vi "Initialize.vi"(6 "Interface":enum16{"RS232", "USB", "Ethernet"}(ring)=enum."USB", 8 "error in (no error)":errorcluster, 9 "reset":bool, 10 "ID query":bool=TRUE, 11 "Address":string) -> (0 "error out":errorcluster, 3 "VISA resource name out":refnum<visa-resource-name>)   [LabVIEW 2016, in "SR7270 Drivers.lvlib" / "SR7270 Drivers.lvclass"]
doc: "This VI passes the addressing information in the instrument decriptor to the Instr Open VI and returns the instrument ID. You can optionally reset the instrument by setting the front panel reset control. You must run this VI before using any of the instrument driver VIs for this instrument.\n\n12 May 2009: First Release"
uses:
  SR7270 Drivers.lvclass
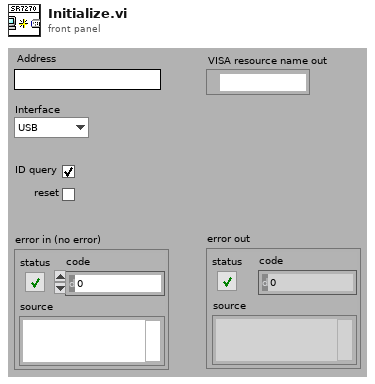
[diagram p1: front panel]
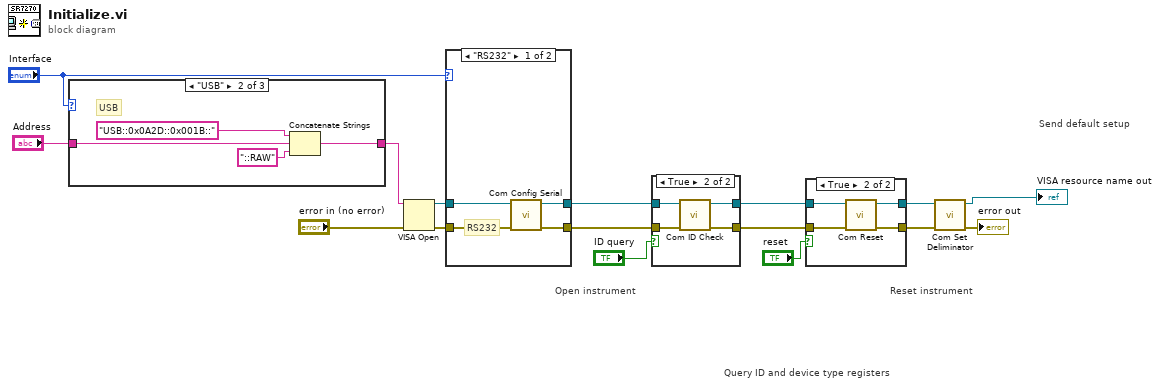
[diagram p0: block diagram]
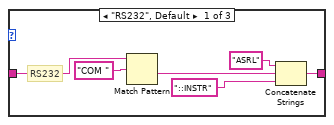
[diagram p5: hidden frame]
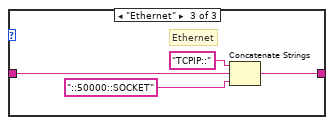
[diagram p6: hidden frame]
diagram:
  # "Send default setup"
  # "Query ID and device type registers"
  # "Reset instrument"
  # "Open instrument"
  n1 = case shown="\"USB\"" "Interface" {
    tunnel: [w22 w26 w30] -> w7
    tunnel: "Address" -> [w19 w23 w27]
    frame "RS232", Default {
      # "RS232"
      n2 = Match Pattern(string=w19, regular expression="COM ") -> (after substring=w20:string)  [unwired: 1 in, 3 out]
      n3 = Concatenate Strings("ASRL", w20, "::INSTR" ("string")) -> (w22:string)
    }
    frame "USB" {
      # "USB"
      n4 = Concatenate Strings("USB::0x0A2D::0x001B::" ("string"), w23, "::RAW" ("string")) -> (w26:string)
    }
    frame "Ethernet" {
      # "Ethernet"
      n5 = Concatenate Strings("TCPIP::" ("string"), w27, "::50000::SOCKET" ("string")) -> (w30:string)
    }
  }
  n6 = VISA Open(error in (no error)="error in (no error)", VISA resource name=w7) -> (VISA resource name=w12:refnum<visa-resource-name>, error out=w10:errorcluster)  [unwired: 3 in]
  n7 = case shown="\"RS232\"" "Interface" {
    tunnel: w12 -> [w34 w36]
    tunnel: [w33 w36] -> w11
    tunnel: w10 -> [w31 w35]
    tunnel: [w32 w35] -> w9
    frame "RS232" {
      # "RS232"
      n8 = call "Com Config Serial.vi"("error in (no error)"=w31, "VISA Refnum in"=w34) -> ("error out"=w32:errorcluster, "VISA Refnum out"=w33:refnum<visa-resource-name>)  [unwired: 8 in]
    }
    frame Default {
    }
  }
  n9 = case shown="True" "ID query" {
    tunnel: [w37 w39] -> w13
    tunnel: [w38 w42] -> w14
    tunnel: w11 -> [w38 w40]
    tunnel: w9 -> [w37 w41]
    frame False {
    }
    frame True {
      n10 = call "Com ID Check.vi"("error in (no error)"=w41, "VISA Refnum in"=w40) -> ("error out"=w39:errorcluster, "VISA Refnum out"=w42:refnum<visa-resource-name>)  [unwired: 8 in]
    }
  }
  n11 = case shown="True" "reset" {
    tunnel: w13 -> [w44 w48]
    tunnel: [w44 w46] -> w6
    tunnel: w14 -> [w43 w47]
    tunnel: [w43 w45] -> w4
    frame False {
    }
    frame True {
      n12 = call "Com Reset.vi"("error in (no error)"=w48, "VISA Refnum in"=w47) -> ("error out"=w46:errorcluster, "VISA Refnum out"=w45:refnum<visa-resource-name>)  [unwired: 8 in]
    }
  }
  n13 = call "Com Set Deliminator.vi"("error in (no error)"=w6, "VISA Refnum in"=w4) -> ("error out"=→"error out":errorcluster, "VISA Refnum out"=→"VISA resource name out":refnum<visa-resource-name>)  [unwired: 8 in]
